vi "Close References.vi"(8 "error in":errorcluster, 11 "Data Subject in":refnum<class "Publisher.lvclass">) -> (0 "error out":errorcluster, 3 "Data Subject out":refnum<class "Publisher.lvclass">)   [LabVIEW 2014, in "Publisher.lvclass"]
doc: "Deallocate the memory for the DVR."
uses:
  Publisher.lvclass
  Publisher.lvclass/Publisher.ctl
  Data/Data.lvclass
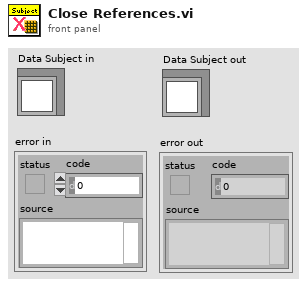
[diagram p1: front panel]
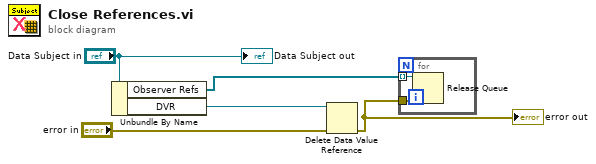
[diagram p0: block diagram]
diagram:
  n1 = Unbundle By Name("Data Subject in") -> ("Observer Refs"=w2:refnum<queue>[], "DVR"=w3:refnum<data-value>)
  n2 = Delete Data Value Reference(data value reference=w3, error in="error in") -> (error out=w1:errorcluster)  [unwired: 1 out]
  "error out" <- w1
  n3 = for {
    tunnel: w2 -> [w7] mode=indexing
    tunnel: w1 -> [w6]
    n4 = Release Queue(queue=w7, error in (no error)=w6) -> ()  [unwired: 1 in, 3 out]
  }
  "Data Subject out" <- "Data Subject in"
